vi "emi_Get Bottom Caller ref if missing.vi"(5 "VI Refnum(Calling VI)":refnum<vi>, 9 "error in (no error)":errorcluster) -> (2 "Ref Generated":bool=TRUE, 6 "VI Refnum Out":refnum<vi>, 10 "error out":errorcluster)   [LabVIEW 2011]
doc: "If VI Refnumis connected to a valid ref number, nothing is done. If it is not, the refnumber of the Bottom caller, teh frst VI in teh app is returned.\n\nThe Idee: help making VIs that default to working with the VI they are placed on. \n\nNo ref number is created if error in."
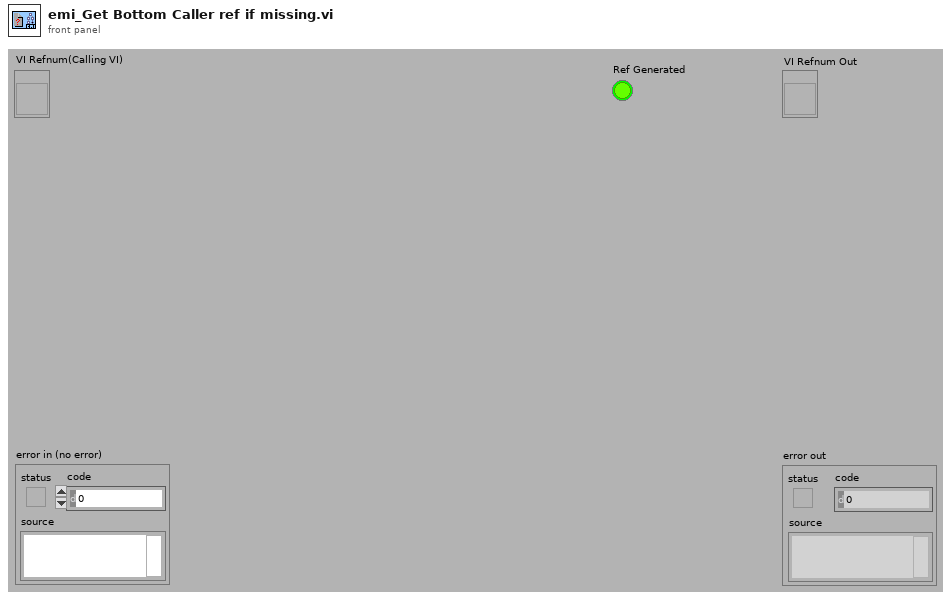
[diagram p1: front panel]
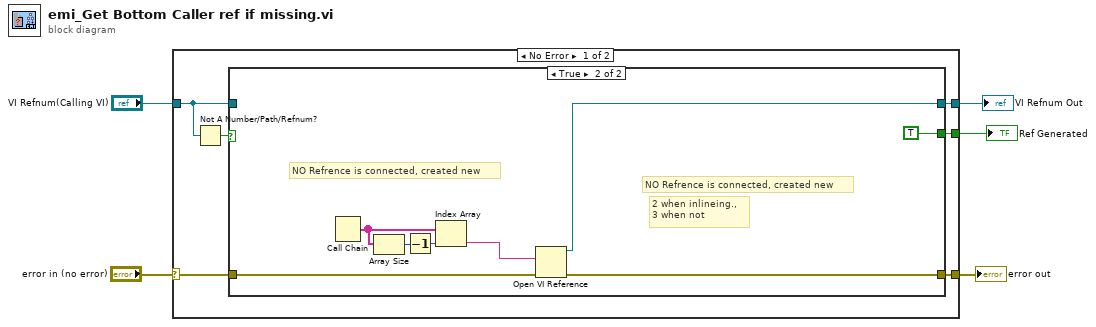
[diagram p0: block diagram]
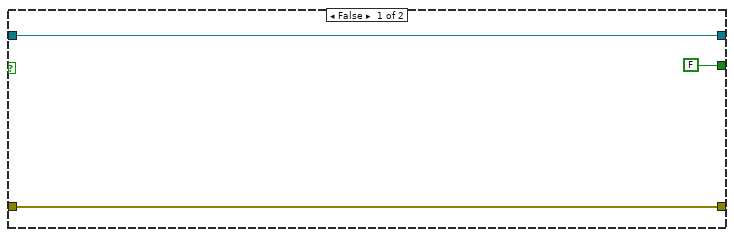
[diagram p2: hidden frame]
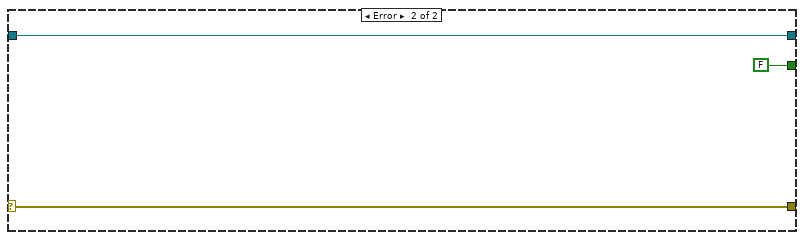
[diagram p3: hidden frame]
diagram:
  n1 = case shown="No Error" "error in (no error)" {
    selector: "error in (no error)" -> [w7 w25]
    tunnel: [w11 w25] -> w5
    tunnel: [w10 w24] -> w4
    tunnel: "VI Refnum(Calling VI)" -> [w8 w24]
    tunnel: [w6 FALSE ("Ref Generated")] -> w1
    frame No Error {
      n2 = Not A Number/Path/Refnum?(number/path/refnum=w8) -> (NaN/Path/Refnum?=w9:bool)
      n3 = case shown="True" w9 {
        tunnel: [w13 w16] -> w11
        tunnel: [w14 w15] -> w10
        tunnel: w8 -> [w14 _]
        tunnel: w7 -> [w13 w17]
        tunnel: [FALSE ("Ref Generated") TRUE ("Ref Generated")] -> w6
        frame False {
        }
        frame True {
          # "2 when inlineing., \n3 when not"
          # "NO Refrence is connected, created new"
          # "NO Refrence is connected, created new"
          n4 = Call Chain() -> (call chain=w20:string[])
          n5 = Array Size(array=w20) -> (size(s)=w21:i32)
          n6 = Decrement(x=w21) -> (x-1=w19:i32)
          n7 = Index Array(array=w20, index=w19) -> (element=w18:string)
          n8 = Open VI Reference(vi path=w18, error in (no error)=w17) -> (vi reference=w15:refnum<vi>, error out=w16:errorcluster)  [unwired: 4 out]
        }
      }
    }
    frame Error {
    }
  }
  "error out" <- w5
  "Ref Generated" <- w1
  "VI Refnum Out" <- w4
